vi "close_front_panel_in_exe.vi"(8 "error_in":errorcluster, 11 "vi_reference_in":refnum<vi>) -> (0 "error_out":errorcluster)   [LabVIEW 2020]
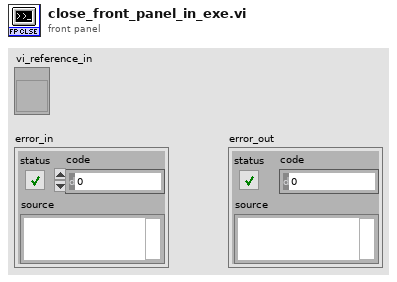
[diagram p1: front panel]
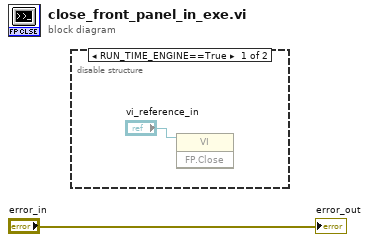
[diagram p0: block diagram]
diagram:
  n1 = disable-structure shown="RUN_TIME_ENGINE==True" {
    frame condition #0 {
      n2 = invoke class="VI" method="FP.Close"(reference="vi_reference_in") -> ()  [unwired: 2 in, 3 out]
    }
    frame condition #1 (active) {
    }
  }
  "error_out" <- "error_in"
